vi "test-linear-filter-test-03A.vi"() -> (3 "Passed":bool)   [LabVIEW 2019]
panel:
  out "Tolerance":dbl
  out "Waveform Graph":dbl[][](graph)
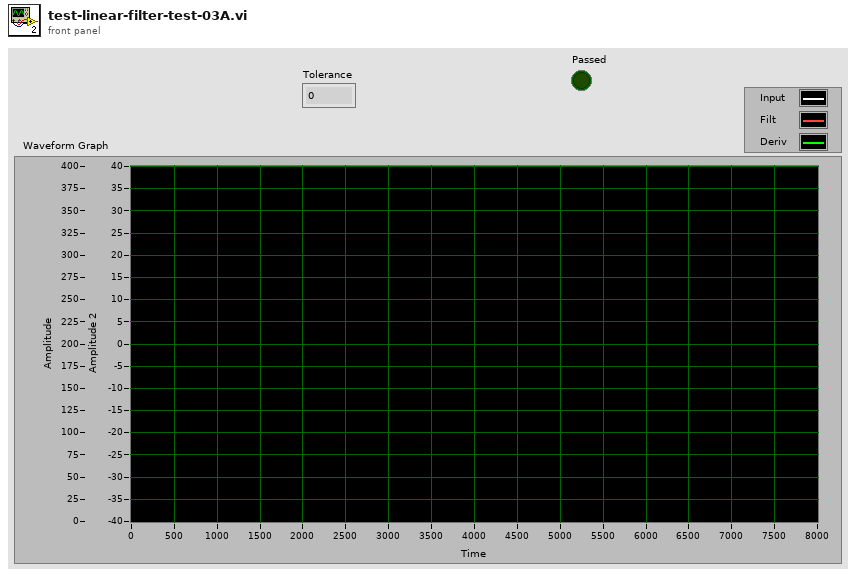
[diagram p1: front panel]
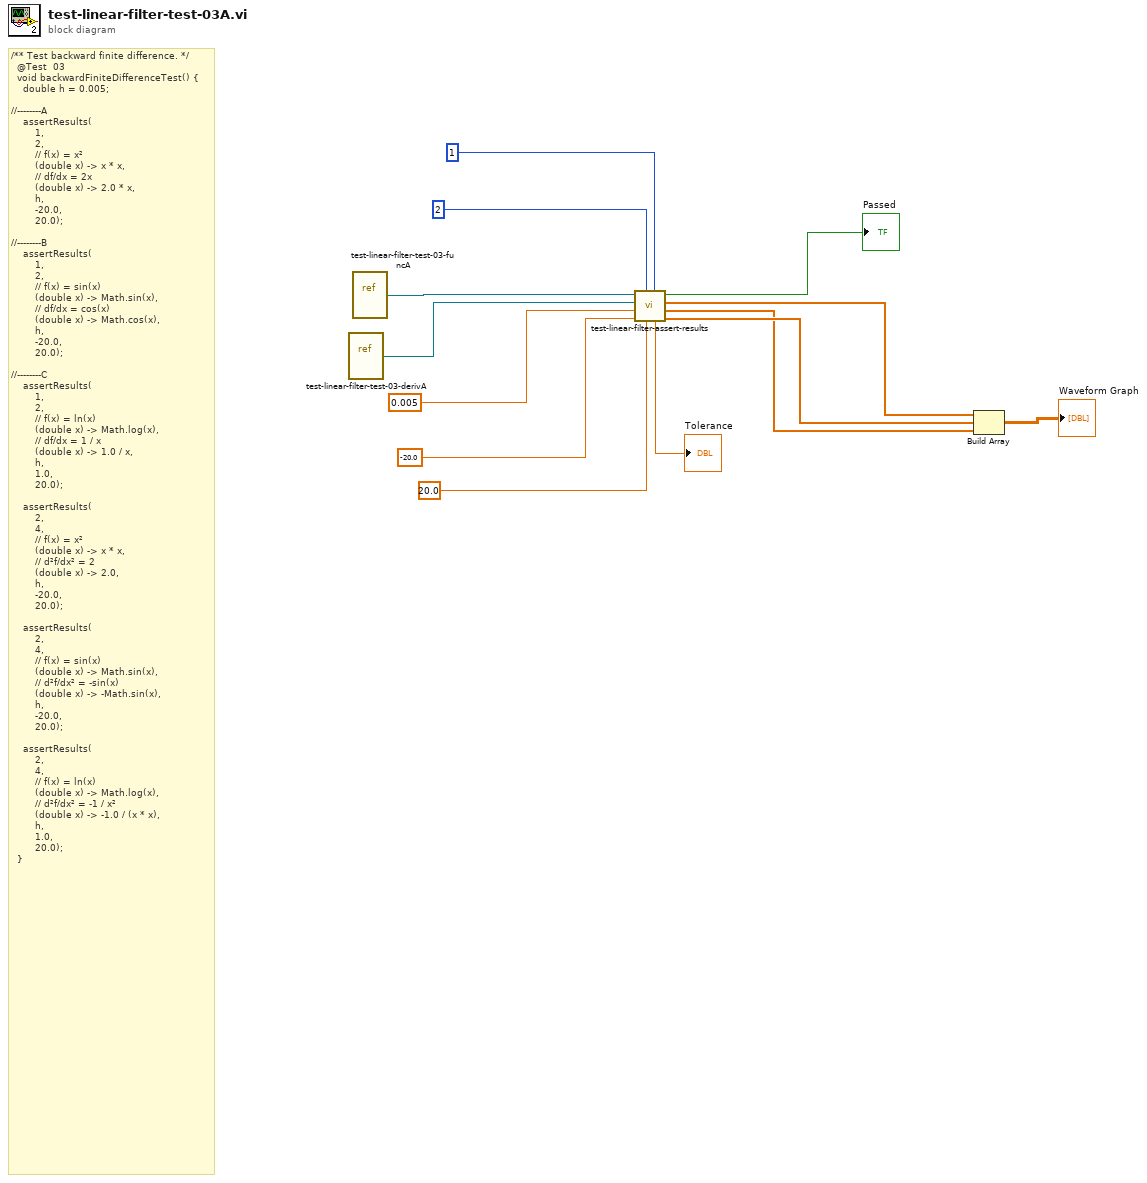
[diagram p0: block diagram]
diagram:
  # "/** Test backward finite difference. */\n  @Test  03\n  void backwardFiniteDifferenceTest() {\n    double h = 0.005;\n\n//--------A\n    assertResults(\n        1,\n        2,\n        // f(x) = x²\n        (double x) -> x * x,\n        // df/dx = 2x\n        (double x) -> 2.0 * x,\n        h,\n        -20.0,\n        20.0);\n\n//--------B\n    assertResults(\n        1,\n        2,\n        // f(x) = sin(x)\n        (double x) -> Math.sin(x),\n        // df/dx = cos(x)\n        (double x) -> Math.cos(x),\n        h,\n        -20.0,\n        20.0);\n\n//--------C\n    assertResults(\n        1,\n        2,\n        // f(x) = ln(x)\n        (double x) -> Math.log(x),\n        // df/dx = 1 / x\n        (double x) -> 1.0 / x,\n        h,\n        1.0,\n        20.0);\n\n    assertResults(\n        2,\n        4,\n        // f(x) = x²\n        (double x) -> x * x,\n        // d²f/dx² = 2\n        (double x) -> 2.0,\n        h,\n        -20.0,\n        20.0);\n\n    assertResults(\n        2,\n        4,\n        // f(x) = sin(x)\n        (double x) -> Math.sin(x),\n        // d²f/dx² = -sin(x)\n        (double x) -> -Math.sin(x),\n        h,\n        -20.0,\n        20.0);\n\n    assertResults(\n        2,\n        4,\n        // f(x) = ln(x)\n        (double x) -> Math.log(x),\n        // d²f/dx² = -1 / x²\n        (double x) -> -1.0 / (x * x),\n        h,\n        1.0,\n        20.0);\n  }"
  n1 = vi-ref "test-linear-filter-test-03-derivA.vi"() -> (w9:refnum<vi>)
  n2 = vi-ref "test-linear-filter-test-03-funcA.vi"() -> (w10:refnum<vi>)
  n3 = call "test-linear-filter-assert-results.vi"("derivative"=1, "Max"=20.0, "Samples"=2, "Min"=-20.0, "H"=0.005, "DerivFunc"=w9, "F"=w10) -> ("Filt"=w4:dbl[], "Deriv"=w1:dbl[], "Raw"=w5:dbl[], "Passed"=→"Passed":bool, "Tolerance"=→"Tolerance":dbl)
  n4 = Build Array(w5, w4, w1) -> (→"Waveform Graph":dbl[][])
